vi "Field measurement.vi"() -> ()   [LabVIEW 2011]
panel:
  out "Temperature Vs. Time":cluster{dbl[], dbl[]}(graph)
  in  "timeout ms (2000)":i32=2000
  out "Time elapsed":string
  in  "Timer":bool caption="Reset"
  in  "date format (0)":enum16{"short", "long", "abbreviated"}(ring)
  in  "Save":bool
  in  "File Path":path
  out "size (in bytes)":i64
  out "Resistance Vs. Temperature":cluster{dbl[], dbl[]}(graph)
  out "Resistance Vs. Field":cluster{dbl[], dbl[]}(graph)
  out "Resistance":string
  out "Temperature":string
  out "Field Vs. Time":cluster{dbl[], dbl[]}(graph)
  out "current time":timestamp
  out "Field (T)":string
  in  "Switch":bool
  in  "Measurement":bool
  in  "error in (no error)":errorcluster
  in  "IP Address":string
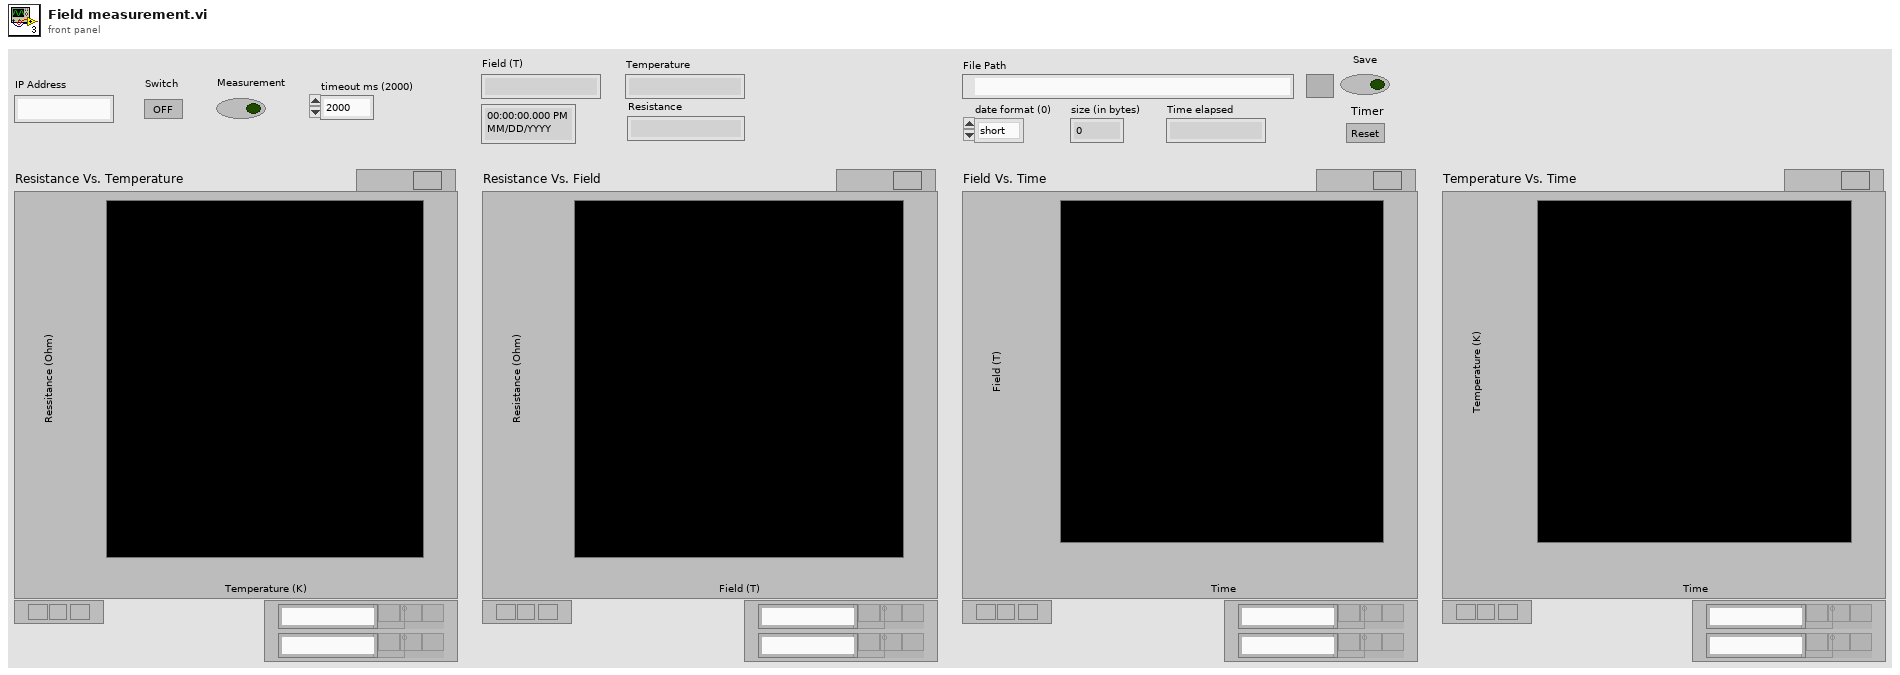
[diagram p1: front panel]
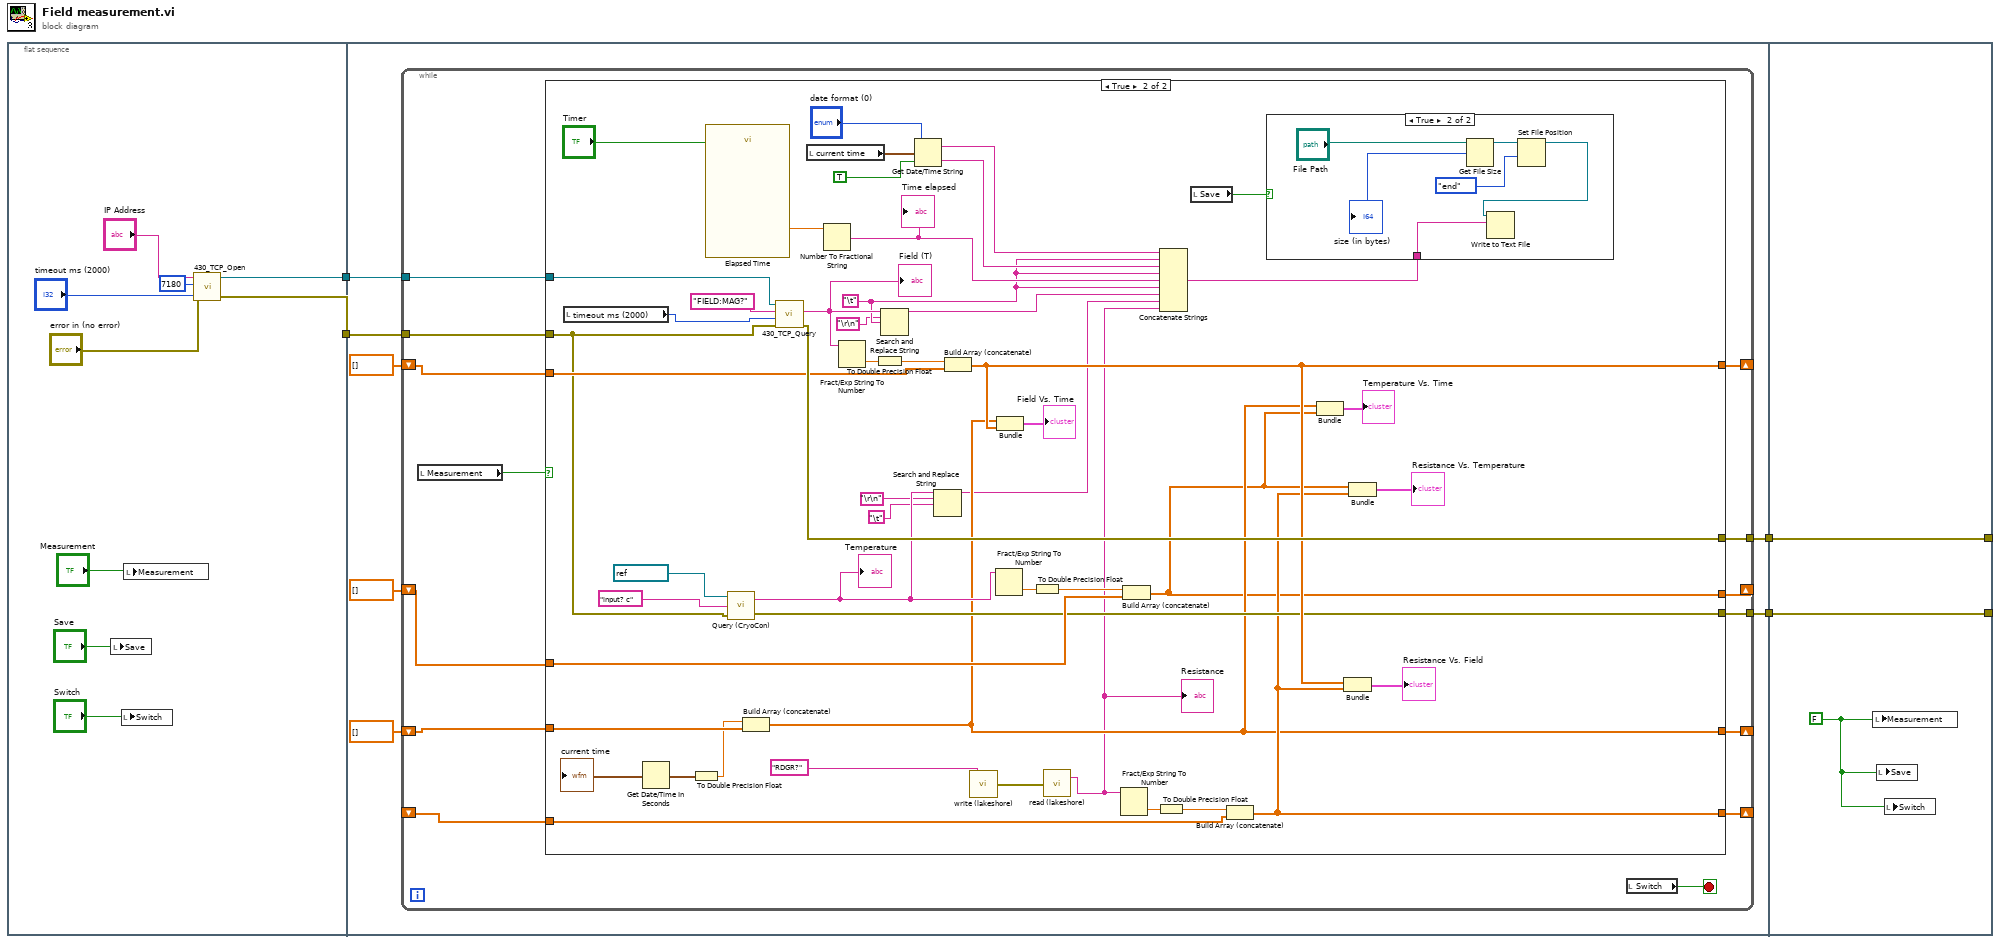
[diagram p0: block diagram]
diagram:
  n1 = flat-sequence {
    tunnel: [w9] -> w4
    tunnel: [w8] -> w3
    tunnel: w4 -> [w20]
    tunnel: w3 -> [w19]
    tunnel: [w18] -> w2
    tunnel: [w15] -> w1
    tunnel: [w96] -> _
    tunnel: [w97] -> _
    tunnel: w2 -> [w97]
    tunnel: w1 -> [w96]
    frame #0 {
      n2 = local write "Save"("Save") -> ()
      n3 = local write "Switch"("Switch") -> ()
      n4 = local write "Measurement"("Measurement") -> ()
      n5 = call "430_TCP_Open.vi"("IP Address"="IP Address", "TCP Port"=7180, "timeout ms (2000)"="timeout ms (2000)", "error in (no error)"="error in (no error)") -> ("connection ID"=w9:refnum<k5>, "error out"=w8:errorcluster)  [unwired: 2 in, 1 out]
    }
    frame #1 {
      n6 = while {
        tunnel: w20 -> [w33]
        tunnel: w19 -> [w32]
        tunnel: [w31] -> w18
        shift-right: [w30] -> _
        shift-left: dbl[] [] -> [w29]
        shift-right: [w28] -> _
        shift-left: dbl[] [] -> [w27]
        tunnel: [w26] -> w15
        shift-right: [w25] -> _
        shift-left: dbl[] [] -> [w24]
        shift-right: [w23] -> _
        shift-left: _ -> [w22]
        stop <- w21 stop-if-true
        n7 = local read "Measurement"() -> (w34:bool)
        n8 = case shown="True" w34 {
          tunnel: w33 -> [_ w87]
          tunnel: w32 -> [w37 w57]
          tunnel: [w37 w86] -> w31
          tunnel: [w38 w47] -> w30
          tunnel: w29 -> [w38 w51]
          tunnel: [w39 w73] -> w28
          tunnel: w27 -> [w39 w83]
          tunnel: [w37 w56] -> w26
          tunnel: [w35 w46] -> w25
          tunnel: w24 -> [w35 w80]
          tunnel: [w36 w48] -> w23
          tunnel: w22 -> [w36 w75]
          frame False {
          }
          frame True {
            w41 = "\t"
            n9 = local read "timeout ms (2000)"() -> (w59:i32)
            n10 = Get Date/Time In Seconds() -> (seconds since 1Jan1904=w85:timestamp)
            "current time" <- w85
            n11 = To Double Precision Float(number=w85) -> (double precision float=w50:dbl)
            n12 = call "Elapsed Time"("Reset"="Timer") -> ("Elapsed Time (s)"=w69:dbl)  [unwired: 11 in, 7 out]
            n13 = call "Query (CryoCon).vi"("error in (no error)"=w57, "write buffer"="input? c", "VISA resource name 2"=refnum<visa-resource-name> "COM3") -> ("error out"=w56:errorcluster, "read buffer"=w54:string)
            "Temperature" <- w54
            n14 = Build Array (concatenate)(w50, w51) -> (w47:dbl[])
            n15 = call "430_TCP_Query.vi"("error in (no error)"=w57, "Timeout"=w59, "Command"="FIELD:MAG?", "connection ID"=w87) -> ("error out"=w86:errorcluster, "Response"=w45:string)  [unwired: 3 in, 3 out]
            "Field (T)" <- w45
            n16 = local read "current time"() -> (w68:timestamp)
            n17 = Number To Fractional String(number=w69) -> (F-format string=w64:string)  [unwired: 3 in]
            "Time elapsed" <- w64
            n18 = Fract/Exp String To Number(string=w45) -> (number=w84:dbl)  [unwired: 3 in, 1 out]
            n19 = To Double Precision Float(number=w84) -> (double precision float=w60:dbl)
            n20 = Search and Replace String(input string=w45, search string="\r\n", replace string=w41) -> (result string=w42:string)  [unwired: 5 in, 3 out]
            n21 = Get Date/Time String(date format (0)="date format (0)", seconds (now)=w68, want seconds? (F)=TRUE) -> (date string=w66:string, time string=w65:string)
            n22 = Search and Replace String(input string=w54, search string="\r\n", replace string="\t") -> (result string=w44:string)  [unwired: 5 in, 3 out]
            n23 = Build Array (concatenate)(w60, w83) -> (w73:dbl[])
            n24 = call "write (lakeshore).vi"("write buffer"="RDGR?") -> ("error out"=w79:errorcluster)  [unwired: 1 in]
            n25 = Fract/Exp String To Number(string=w54) -> (number=w81:dbl)  [unwired: 3 in, 1 out]
            n26 = Bundle(w47, w73) -> (→"Field Vs. Time":cluster{dbl[], dbl[]})  [unwired: 1 in]
            n27 = To Double Precision Float(number=w81) -> (double precision float=w61:dbl)
            n28 = call "read (lakeshore).vi"("error in (no error)"=w79) -> ("read buffer"=w43:string)  [unwired: 1 out]
            "Resistance" <- w43
            n29 = Fract/Exp String To Number(string=w43) -> (number=w77:dbl)  [unwired: 3 in, 1 out]
            n30 = Build Array (concatenate)(w61, w80) -> (w46:dbl[])
            n31 = To Double Precision Float(number=w77) -> (double precision float=w76:dbl)
            n32 = Concatenate Strings(w66, w41, w65, w41, w64, w41, w42, w44, w43) -> (w71:string)
            n33 = local read "Save"() -> (w70:bool)
            n34 = Build Array (concatenate)(w76, w75) -> (w48:dbl[])
            n35 = case shown="True" w70 {
              tunnel: w71 -> [_ w94]
              frame False {
              }
              frame True {
                n36 = Get File Size(file="File Path") -> (refnum out=w92:refnum<file>, size (in bytes)=→"size (in bytes)":i64)  [unwired: 1 in, 1 out]
                n37 = Set File Position(refnum=w92, from (0:start)=enum16{"start", "end", "current"}."end") -> (refnum out=w91:refnum<file>)  [unwired: 2 in, 1 out]
                n38 = Write to Text File(file (use dialog)=w91, text=w94) -> ()  [unwired: 2 in, 3 out]
              }
            }
            n39 = Bundle(w47, w46) -> (→"Temperature Vs. Time":cluster{dbl[], dbl[]})  [unwired: 1 in]
            n40 = Bundle(w73, w48) -> (→"Resistance Vs. Field":cluster{dbl[], dbl[]})  [unwired: 1 in]
            n41 = Bundle(w46, w48) -> (→"Resistance Vs. Temperature":cluster{dbl[], dbl[]})  [unwired: 1 in]
          }
        }
        n42 = local read "Switch"() -> (w21:bool)
      }
    }
    frame #2 {
      w95 = FALSE ("Measurement")
      n43 = local write "Measurement"(w95) -> ()
      n44 = local write "Save"(w95) -> ()
      n45 = local write "Switch"(w95) -> ()
    }
  }
